vi "4-6 ForLoopSum.vi"() -> ()   [LabVIEW 2014]
doc: "------------------------------------\nAuther: Koji Ohashi\nCopyright (c) 2020 Japan LabVIEW Users Group, Volunteer members.\nThis VI is released under the MIT License.\nhttp://opensource.org/licenses/mit-license.php\n------------------------------------"
panel:
  out "Final value of calculation":i32
  out "Array of shift register output":i32[](array[numeric])
  out "Array of iteration terminal value":i32[](array[numeric])
  out "Array of additional value":i32[](array[numeric])
  out "Array of calculation progress (input to shift register)":i32[](array[numeric])
  out "Total value from 1 to N":i32
  in  "N":i32=10
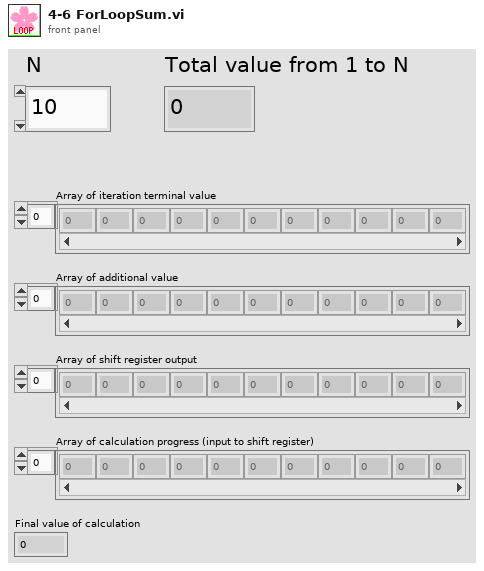
[diagram p1: front panel]
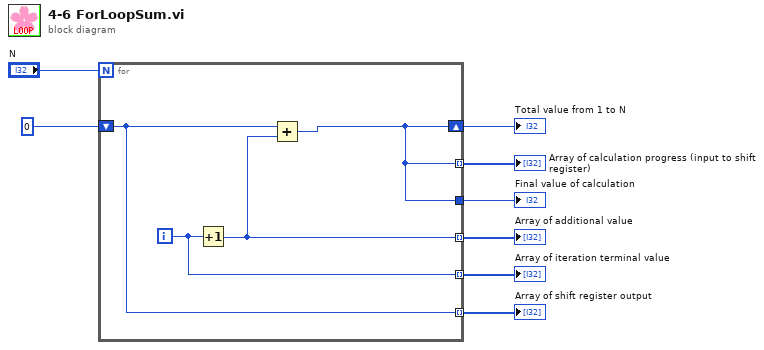
[diagram p0: block diagram]
diagram:
  n1 = for {
    N: "N" -> [_]
    shift-right: [w9] -> w8
    shift-left: 0 -> [w10]
    tunnel: [w9] -> w7 mode=indexing
    tunnel: [w12] -> w6 mode=indexing
    tunnel: [w11] -> w5 mode=indexing
    tunnel: [w10] -> w4 mode=indexing
    tunnel: [w9] -> w3
    i -> [w11]
    n2 = Increment(x=w11) -> (x+1=w12:i32)
    n3 = Add(x=w10, y=w12) -> (x+y=w9:i32)
  }
  "Total value from 1 to N" <- w8
  "Array of calculation progress (input to shift register)" <- w7
  "Array of additional value" <- w6
  "Array of iteration terminal value" <- w5
  "Array of shift register output" <- w4
  "Final value of calculation" <- w3
